vi "Save Data.vi"(6 "Data save config":T1={"Filename"="", "Comment"="", "Enable"=TRUE, "Filepath"=path ""}, 8 "error in":errorcluster, 9 "Timestamp":string, 10 "File type":string, 11 "data":waveform(dbl)[](array[waveform])) -> (0 "error out":errorcluster, 3 "appended path":path)   [LabVIEW 2019]
panel:
  # "Save waveform data"
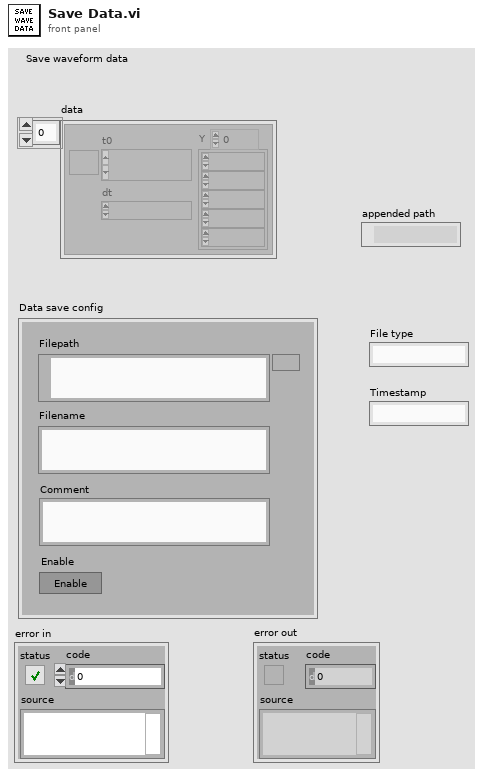
[diagram p1: front panel]
types:
  T1 = cluster{"Filename":string, "Comment":string, "Enable":bool, "Filepath":path}
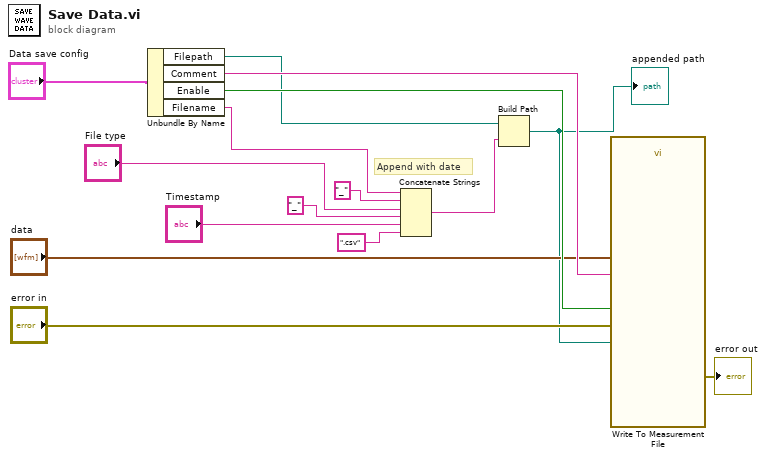
[diagram p0: block diagram]
diagram:
  # "Append with date"
  n1 = Unbundle By Name("Data save config") -> ("Filepath"=w8:path, "Comment"=w12:string, "Enable"=w13:bool, "Filename"=w5:string)
  n2 = Concatenate Strings(w5, "_" ("string"), "File type", "_" ("string"), "Timestamp", ".csv" ("string")) -> (w9:string)
  n3 = Build Path(base path=w8, name or relative path=w9) -> (appended path=w7:path)
  "appended path" <- w7
  n4 = call "Write To Measurement File"("Signals"="data", "Enable"=w13, "error in (no error)"="error in", "Filename"=w7, "Comment"=w12) -> ("error out"=→"error out":errorcluster)  [unwired: 12 in, 2 out]
